vi "Test bench.vi"() -> ()   [LabVIEW 2013]
uses:
  <vilib>/rvi/DesktopExecutionNode/Execution/niFpgaDEN_Execute.vi
  <vilib>/Utility/file.llb/Write To Spreadsheet File (I64).vi
  <vilib>/rvi/DesktopExecutionNode/DesktopExecutionNode.xnode
panel:
  out "AI Raw":u32
  in  "file path (dialog if empty)":path
  in  "StreamToDMA":bool
  in  "SamplingEnable":bool
  in  "stop":bool
  out "LedIndex":u32
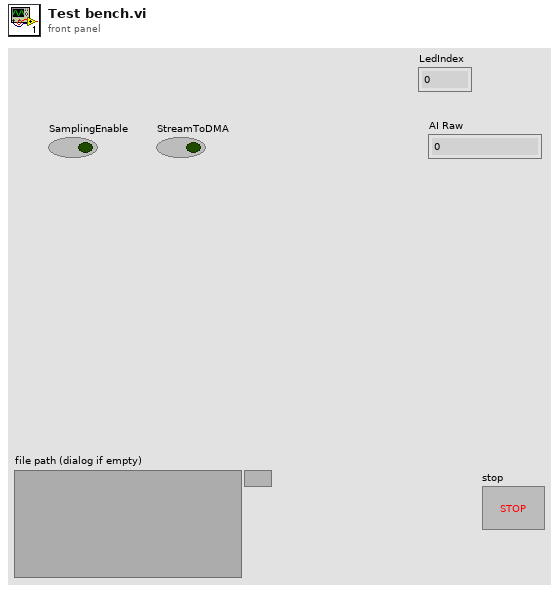
[diagram p1: front panel]
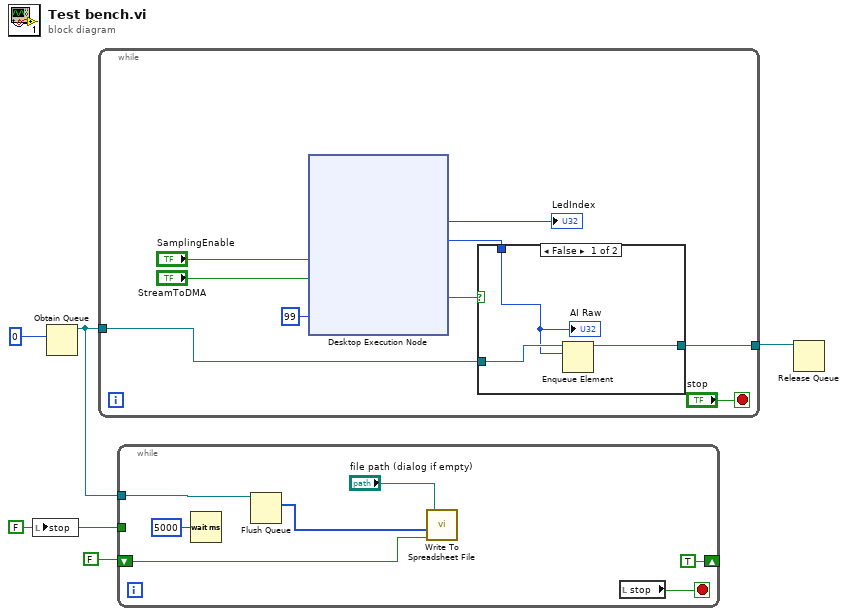
[diagram p0: block diagram]
diagram:
  w1 = FALSE ("stop")
  n1 = local write "stop"(w1) -> ()
  n2 = Obtain Queue(element data type=u32 0) -> (queue out=w3:refnum<queue>)  [unwired: 4 in, 2 out]
  n3 = while {
    tunnel: w3 -> [w8]
    tunnel: [w7] -> w4
    stop <- "stop" stop-if-true
    n4 = xnode "Desktop Execution Node"("SamplingEnable"="SamplingEnable", "StreamToDMA"="StreamToDMA", "SampPerPulse"=u8 99) -> ("LedIndex"=→"LedIndex":u32, "AI Raw"=w13:u32, "RawFifoWrite"=w9:bool)  [unwired: 1 in, 1 out]
    n5 = case shown="False" w9 {
      tunnel: w13 -> [w15 _]
      tunnel: w8 -> [w17 w18]
      tunnel: [w16 w18] -> w7
      frame False {
        n6 = Enqueue Element(queue=w17, element=w15) -> (queue out=w16:refnum<queue>)  [unwired: 2 in, 2 out]
        "AI Raw" <- w15
      }
      frame True {
      }
    }
  }
  n7 = while {
    tunnel: w3 -> [w20]
    shift-right: [TRUE] -> _
    shift-left: FALSE -> [w23]
    tunnel: w1 -> [_]
    stop <- w21 stop-if-true
    n8 = Wait (ms)(milliseconds to wait=u32 5000) -> ()  [unwired: 1 out]
    n9 = Flush Queue(queue=w20) -> (remaining elements=w19:u32[])  [unwired: 1 in, 2 out]
    n10 = call-poly <vilib>:"Write To Spreadsheet File.vi"("append to file? (new file:F)"=w23, "1D data"=w19, "file path (dialog if empty)"="file path (dialog if empty)") -> ()  [unwired: 5 in, 1 out]
    n11 = local read "stop"() -> (w21:bool)
  }
  n12 = Release Queue(queue=w4) -> ()  [unwired: 2 in, 3 out]
